vi "Close.vi"(8 "error in (no error)":errorcluster, 11 "Data in":refnum<class "Const_CPLX_EXT.lvclass">) -> (0 "error out":errorcluster, 3 "Data out":refnum<class "Const_CPLX_EXT.lvclass">)   [LabVIEW 2021, in "Const_CPLX_EXT.lvclass"]
uses:
  Const_CPLX_EXT.lvclass
  Abs_Types/Complex Extended Float/Abs_Complex Extended Float.lvclass
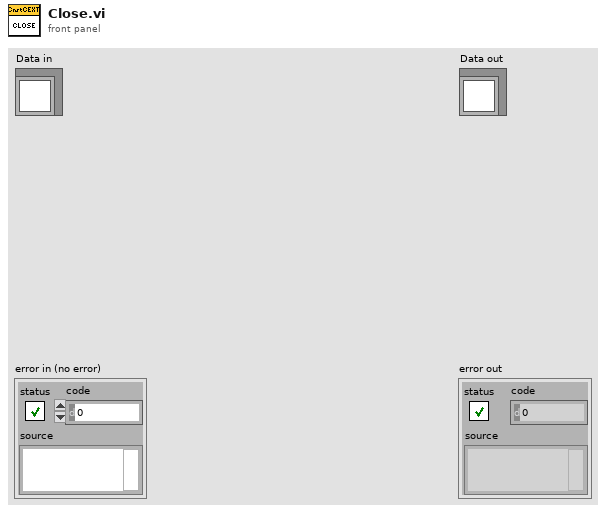
[diagram p1: front panel]
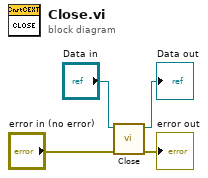
[diagram p0: block diagram]
diagram:
  n1 = call-parent "Close.vi"("error in (no error)"="error in (no error)", "Data in"="Data in") -> ("error out"=→"error out":errorcluster, "Data out"=→"Data out":refnum<class "Const_CPLX_EXT.lvclass">)  [unwired: 8 in]
